vi "Bind To Name.vi"(8 "error in (no error)":errorcluster, 10 "Type":refnum<class>, 11 "Serialization Binder in":refnum<class "Serialization Binder.lvclass">) -> (0 "error out":errorcluster, 2 "Type Name":string, 3 "Serialization Binder out":refnum<class "Serialization Binder.lvclass">)   [LabVIEW 2017, in "Serialization Binder.lvclass"]
doc: "Controls the binding of a type to a serialized object."
uses:
  Serialization Binder.lvclass
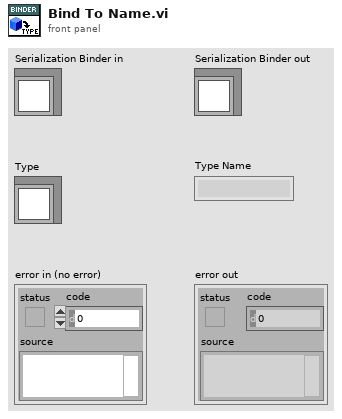
[diagram p1: front panel]
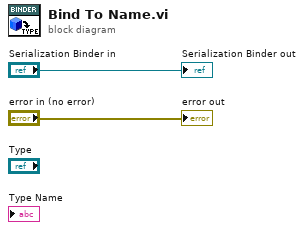
[diagram p0: block diagram]
diagram:
  "error out" <- "error in (no error)"
  "Serialization Binder out" <- "Serialization Binder in"
